vi "0805_Visão_de_máquina_alterado.vi"() -> ()   [LabVIEW 2017]
uses:
  <vilib>/userdefined/High Color/IMAQdx.ctl
  <vilib>/vision/driver/IMAQdx.llb/IMAQdx Acquisition Mode.ctl
  <vilib>/vision/driver/IMAQdx.llb/IMAQdx Buffer Number Mode.ctl
  <vilib>/vision/Classification.llb/IMAQ Classifier Read Options.ctl
  <vilib>/vision/driver/NI_Vision_Acquisition_Software.lvlib
  <vilib>/vision/NI_Vision_Development_Module.lvlib
panel:
  out "String":string="Vermelho"
  in  "largura_y":sgl=30.0
  in  "largura_x":sgl=30.0
  in  "ofset y":sgl
  in  "ofset x":sgl
  out "Local destino":T1(ring)
  in  "Tab Control":T2(tab)
  in  "Cluster A":T3
  in  "Cluster B":T3
  in  "Cluster C":T3
  in  "QRCode":bool
  out "Table":string[][](table)
  in  "Stop 2":bool
  in  "Stop 1":bool
  out "Imagem Original":T4(plugin-control)
  in  "Câmera":T5="cam1"
  out "XY Graph 2":cluster{"X":dbl, "Y":dbl}[](graph)
  # "0"
  # "-250"
  # "400"
  # "80"
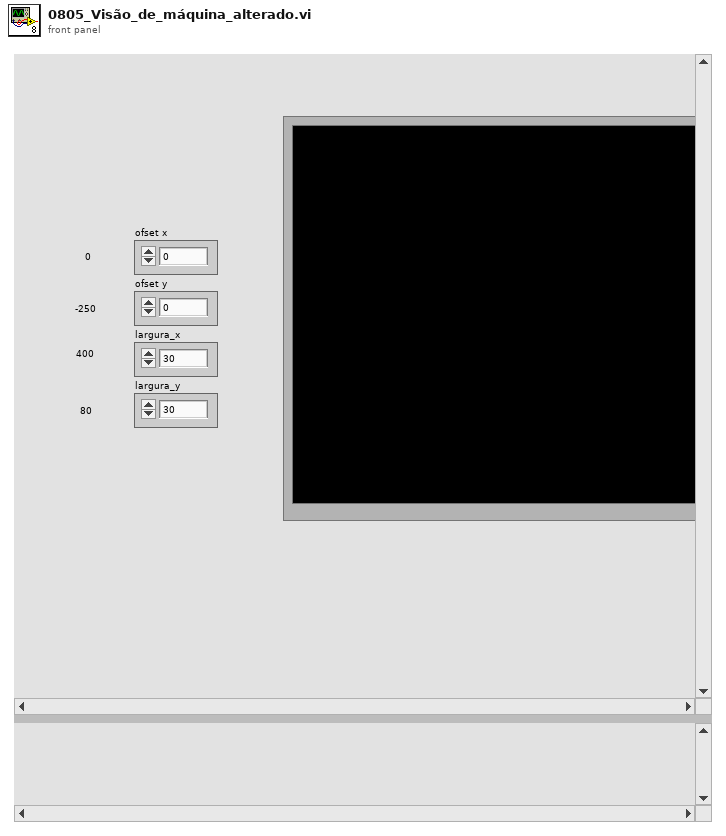
[diagram p1: front panel]
types:
  T1 = enum16{"Local A", "Local B", "Local C", "Discard"}
  T2 = enum32{"Local A", "Local B", "Local C", "QRCode"}
  T3 = cluster{"Azul":bool, "Verde":bool, "Vermelho":bool, "Amarelo":bool, "Quadrado":bool, "Triângulo":bool, "Trapézio":bool}
  T4 = typedef "IMAQ Image.ctl" = refnum<image>
  T5 = typedef "IMAQdx.ctl" = refnum<k21>
  T6 = typedef "NI_Vision_Acquisition_Software.lvlib/IMAQdx Acquisition Mode.ctl" = enum32{"One Shot", "Continuous"}
  T7 = typedef "NI_Vision_Acquisition_Software.lvlib/IMAQdx Buffer Number Mode.ctl" = enum32{"Next", "Last", "Buffer Number", "Every", "Last New"}
  T8 = cluster{"Global Rectangle":i32[], "Contours":cluster{"Contour Type":u32, "ROI Type":u32, "Points":i32[]}[]}
  T9 = typedef "ROI Descriptor" = cluster{"Global Rectangle":i32[], "Contours":cluster{"ID":enum32{"External", "Internal"}, "Type":u32, "Coordinates":i32[]}[]}
  T10 = typedef "IMAQ Classifier Read Options.ctl" = i32
  T11 = typedef "IMAQ Classifier Session.ctl" = refnum<k1>
  T12 = cluster{"Contour Type":u32, "ROI Type":u32, "Points":i32[]}[]
  T13 = cluster{"Contour Type":u32, "ROI Type":u32, "Points":i32[]}
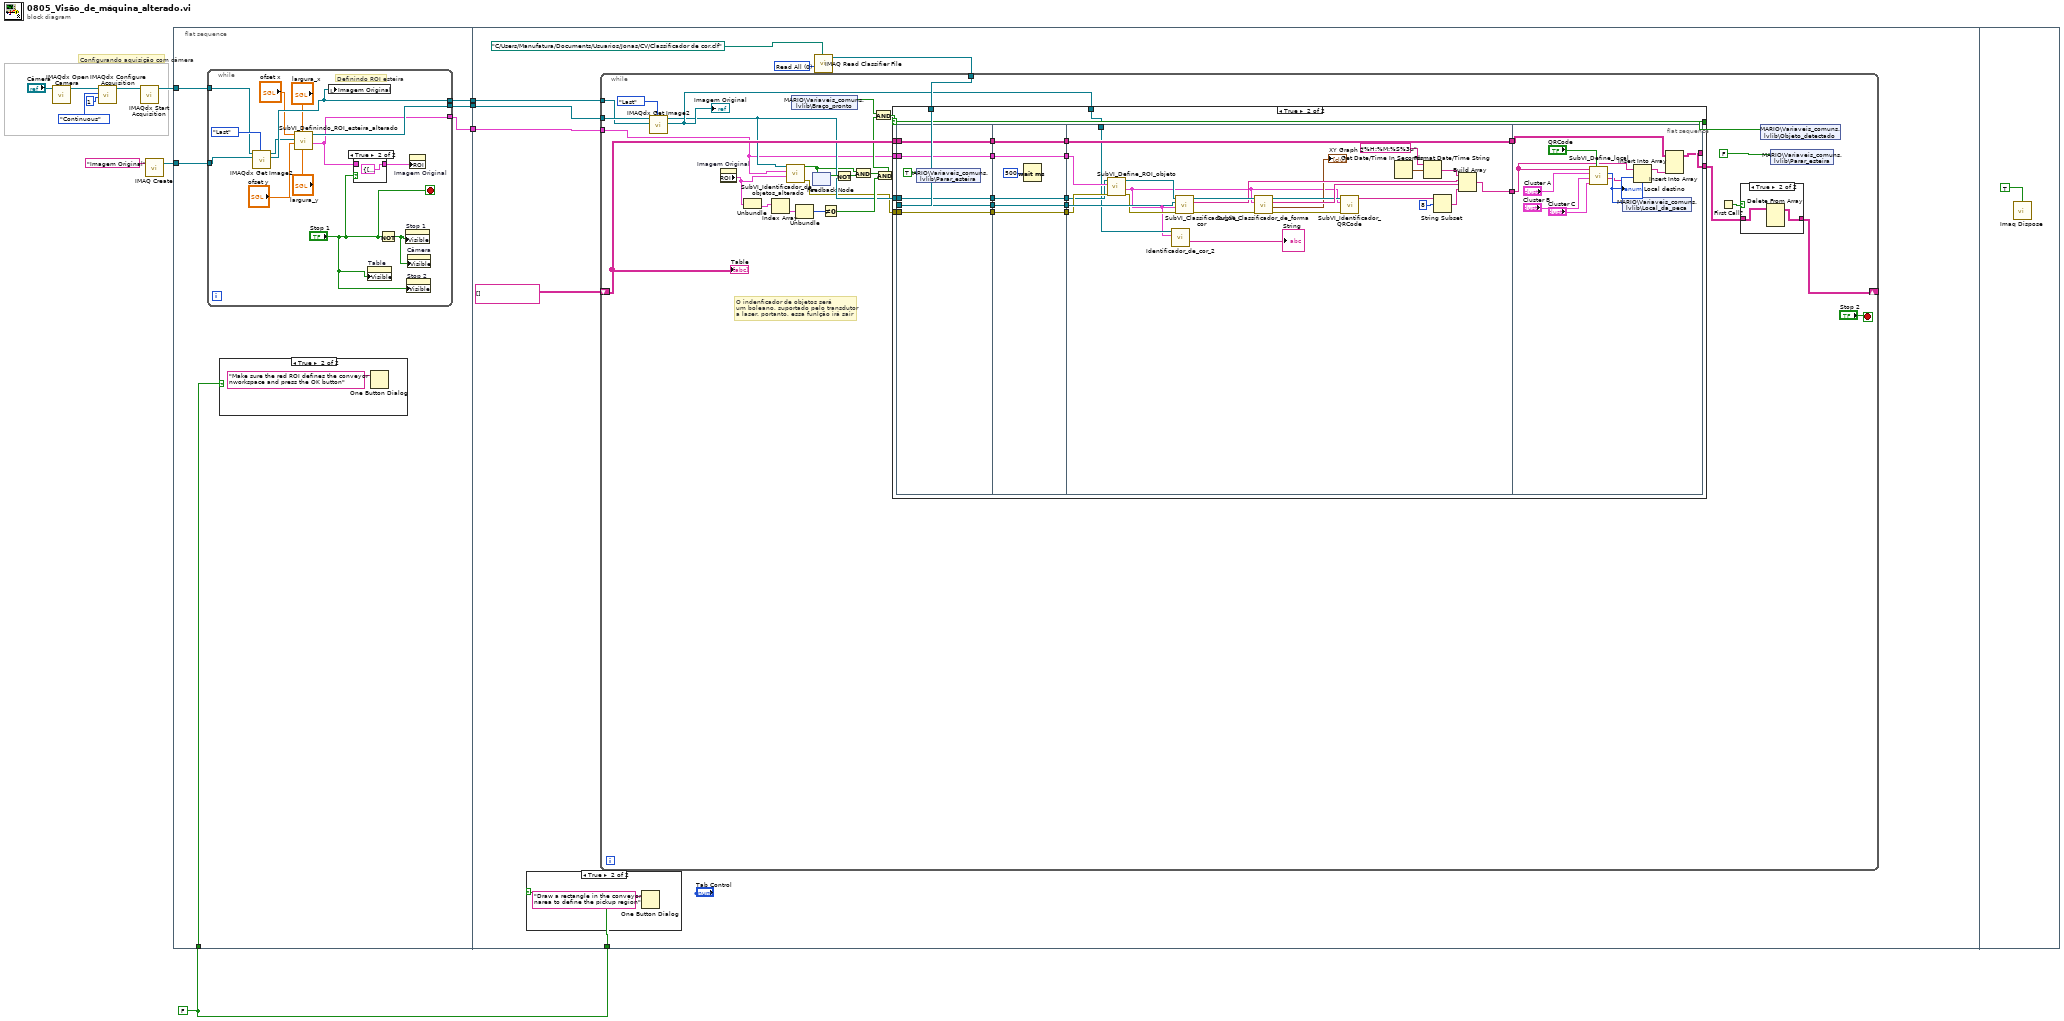
[diagram p0: block diagram]
diagram:
  w1 = FALSE
  # "Configurando aquisição com câmera"
  n1 = call <vilib>:"IMAQdx Open Camera.vi"("Session In"="Câmera") -> ("Session Out"=w12:T5)  [unwired: 9 in, 1 out]
  n2 = call <vilib>:"IMAQdx Configure Acquisition.vi"("Number of Buffers"=u32 1, "Continuous?"=IMAQdx_Acquisition_Mode."Continuous", "Session In"=w12) -> ("Session Out"=w11:T5)  [unwired: 7 in, 1 out]
  n3 = call <vilib>:"IMAQdx Start Acquisition.vi"("Session In"=w11) -> ("Session Out"=w7:T5)  [unwired: 9 in, 1 out]
  n4 = call "IMAQ Create"("Image Name"="Imagem Original") -> ("New Image"=w5:T4)  [unwired: 4 in, 1 out]
  n5 = flat-sequence {
    tunnel: w7 -> [w18]
    tunnel: w5 -> [w17]
    tunnel: [w16] -> w4
    tunnel: [w15] -> w3
    tunnel: [w14] -> w2
    tunnel: w1 -> [w13]
    tunnel: w4 -> [w43]
    tunnel: w3 -> [w42]
    tunnel: w2 -> [w41]
    tunnel: w1 -> [w40]
    frame #0 {
      n6 = while {
        tunnel: w18 -> [w32]
        tunnel: w17 -> [w31]
        tunnel: [w25] -> w16
        tunnel: [w24] -> w15
        tunnel: [w29] -> w14
        stop <- "Stop 1" stop-if-true
        # "Definindo ROI esteira"
        n7 = call <vilib>:"IMAQdx Get Image2.vi"("Buffer Number Mode (Next)"=IMAQdx_Buffer_Number_Mode."Last", "Image In"=w31, "Session In"=w32) -> ("Image Out"=w29:T4, "Session Out"=w26:T5)  [unwired: 5 in, 2 out]
        n8 = call "SubVI_Definindo_ROI_esteira_alterado.vi"("largura_y"="largura_y", "largura_x"="largura_x", "ofset y"="ofset y", "Session in"=w26, "ofset x"="ofset x") -> ("ROI Descriptor"=w24:T9, "Session Out"=w25:T5)  [unwired: 4 in, 1 out]
        n9 = local write "Imagem Original"(w29) -> ()
        n10 = case shown="True" "Stop 1" {
          tunnel: w24 -> [w34 _]
          tunnel: [w34 T8 {"Global Rectangle"=[0, 0, 1, 1], "Contours"=[{"Contour Type"=0, "ROI Type"=1, "Points"=[0, 0]}]} ("ROI")] -> w30
          frame False {
          }
          frame True {
          }
        }
        n11 = property on="Table" class="Tbl (strict)"("Visible"="Stop 1") -> ()  [unwired: 2 in, 2 out]
        n12 = Not(x="Stop 1") -> (.not. x?=w28:bool)
        n13 = property on="Stop 1" class="Bool"("Visible"=w28) -> ()  [unwired: 2 in, 2 out]
        n14 = property on="Stop 2" class="Bool"("Visible"="Stop 1") -> ()  [unwired: 2 in, 2 out]
        n15 = property on="Câmera" class="IMAQdx (strict)"("Visible"=w28) -> ()  [unwired: 2 in, 2 out]
        n16 = property on="Imagem Original" class="ImageControl"("ROI"=w30) -> ()  [unwired: 2 in, 2 out]
      }
      n17 = case shown="True" w13 {
        frame False {
        }
        frame True {
          n18 = One Button Dialog(message="Make sure the red ROI defines the conveyor \nworkspace and press the OK button") -> ()  [unwired: 1 in, 1 out]
        }
      }
    }
    frame #1 {
      w39 = T10 0 items=["Read All", "Add Samples, Do Not Change Options", "Read Options, Do Not Add Samples"] ("Read Options")
      n19 = case shown="True" w40 {
        frame False {
        }
        frame True {
          n20 = One Button Dialog(message="Draw a rectangle in the conveyor\narea to define the pickup region") -> ()  [unwired: 1 in, 1 out]
        }
      }
      n21 = call "IMAQ Read Classifier File"("File Path"=path "C:/Users/Manufatura/Documents/Usuarios/Jonas/CV/Classificador de cor.clf", "Read Options"=w39) -> ("Classifier Session"=w38:T11)  [unwired: 2 in, 7 out]
      n22 = while {
        tunnel: w43 -> [w69]
        tunnel: w42 -> [w47]
        tunnel: w41 -> [w67]
        tunnel: w38 -> [w62]
        shift-right: [w55] -> _
        shift-left: string[][] [] ("Table") -> [w58]
        stop <- "Stop 2" stop-if-true
        # "O indenficador de objetos será\num boleano, suportado pelo transdutor\na laser. portanto, essa funlção irá sair"
        n23 = call <vilib>:"IMAQdx Get Image2.vi"("Buffer Number Mode (Next)"=IMAQdx_Buffer_Number_Mode."Last", "Image In"=w67, "Session In"=w69) -> ("Image Out"=w49:T4, "Session Out"=w48:T5)  [unwired: 5 in, 2 out]
        "Imagem Original" <- w49
        n24 = property on="Imagem Original" class="ImageControl"() -> ("ROI"=w46:T8)  [unwired: 2 in, 2 out]
        n25 = Unbundle(w46) -> ("Contours"=w66:T12)  [unwired: 1 out]
        n26 = Index Array(array=w66) -> (element=w65:T13)  [unwired: 1 in]
        n27 = call "SubVI_Identificador_de_objetos_alterado.vi"("ROI Detecção"=w46, "ROI Esteira"=w47, "Session In"=w48) -> ("error out"=w44:errorcluster, "Objeto Identificado"=w45:bool)  [unwired: 7 in]
        n28 = shared-variable "MARIO\\Variaveis_comuns.lvlib\\Braço_pronto"() -> (w52:bool)  [unwired: 1 in, 1 out]
        n29 = Unbundle(w65) -> ("ROI Type"=w64:u32)  [unwired: 2 out]
        n30 = feedback-in #1(w45) -> ()
        n31 = feedback #1() -> (w60:bool)  [unwired: 1 in]
        n32 = Not Equal To 0?(x=w64) -> (x != 0?=w63:bool)
        n33 = Not(x=w60) -> (.not. x?=w59:bool)
        n34 = And(x=w45, y=w59) -> (x .and. y?=w61:bool)
        n35 = And(x=w61, y=w63) -> (x .and. y?=w51:bool)
        n36 = And(x=w52, y=w51) -> (x .and. y?=w50:bool)
        n37 = case shown="True" w50 {
          selector: w50 -> [w74 w89]
          tunnel: w48 -> [_ w93]
          tunnel: w62 -> [_ w95]
          tunnel: w44 -> [_ w94]
          tunnel: [w75 w92] -> w56
          tunnel: w58 -> [w75 w91]
          tunnel: [w74 w89] -> w54
          tunnel: w47 -> [_ w88]
          tunnel: w49 -> [_ w76]
          frame False {
          }
          frame True {
            n38 = flat-sequence {
              tunnel: w91 -> [w98]
              tunnel: w93 -> [w99]
              tunnel: w94 -> [w100]
              tunnel: w95 -> [w101]
              tunnel: [w101] -> w87
              tunnel: [w100] -> w85
              tunnel: [w99] -> w83
              tunnel: [w98] -> w81
              tunnel: w88 -> [w96]
              tunnel: [w96] -> w79
              tunnel: w87 -> [w107]
              tunnel: [w107] -> w86
              tunnel: w85 -> [w106]
              tunnel: [w106] -> w84
              tunnel: w83 -> [w105]
              tunnel: [w105] -> w82
              tunnel: w81 -> [w104]
              tunnel: [w104] -> w80
              tunnel: w79 -> [w103]
              tunnel: [w103] -> w78
              tunnel: [w119] -> w90
              tunnel: w86 -> [w131]
              tunnel: w84 -> [w116]
              tunnel: w82 -> [w114]
              tunnel: w80 -> [w113]
              tunnel: w78 -> [w117]
              tunnel: [w113] -> w77
              tunnel: w76 -> [w109]
              tunnel: [w135] -> w92
              tunnel: w90 -> [w134]
              tunnel: w77 -> [w136]
              frame #0 {
                n39 = shared-variable "MARIO\\Variaveis_comuns.lvlib\\Parar_esteira"(TRUE ("Parar_esteira")) -> ()  [unwired: 1 in, 1 out]
              }
              frame #1 {
                n40 = Wait (ms)(milliseconds to wait=u32 500) -> ()  [unwired: 1 out]
              }
              frame #2 {
                n41 = call "SubVI_Define_ROI_objeto.vi"("error in (no error)"=w116, "ROI Esteira"=w117, "Session In"=w114) -> ("error out"=w115:errorcluster, "ROI Objeto"=w108:T9, "Session Out"=w110:T5)  [unwired: 5 in, 1 out]
                n42 = call "Identificador_de_cor_2.vi"("ROI Objeto"=w108, "Refnum in"=w109) -> ("String"=→"String":string)  [unwired: 6 in, 3 out]
                n43 = call "SubVI_Classificador_de_cor.vi"("error in"=w115, "ROI Objeto"=w108, "Classifier Session"=w131, "Session In"=w110) -> ("error out"=w130:errorcluster, "Class"=w118:string, "Session Out"=w125:T5)  [unwired: 5 in]
                n44 = call "SubVI_Classificador_de_forma.vi"("error in"=w130, "ROI Objeto"=w108, "Session In"=w125) -> ("error out"=w126:errorcluster, "Points"=→"XY Graph 2":cluster{"X":dbl, "Y":dbl}[], "Forma"=w124:string, "Session Out"=w123:T5)  [unwired: 5 in]
                n45 = call "SubVI_Identificador_QRCode.vi"("error in"=w126, "ROI Objeto"=w108, "Session In"=w123) -> ("Data"=w122:string)  [unwired: 7 in, 1 out]
                n46 = Get Date/Time In Seconds() -> (seconds since 1Jan1904=w128:timestamp)
                n47 = Format Date/Time String(time format string (%c)="%H:%M:%S%3u", seconds (now)=w128) -> (date/time string=w127:string)  [unwired: 1 in]
                n48 = String Subset(string=w122, offset (0)=8) -> (substring=w121:string)  [unwired: 1 in]
                n49 = Build Array(w127, w118, w124, w121) -> (w119:string[])
              }
              frame #3 {
                n50 = call "SubVI_Define_local.vi"("QRCode"="QRCode", "Cluster C"="Cluster C", "Cluster B"="Cluster B", "Cluster A"="Cluster A", "Linha da tabela"=w134) -> ("Destino"=w132:string, "Local destino"=w138:T1)  [unwired: 5 in]
                "Local destino" <- w138
                n51 = shared-variable "MARIO\\Variaveis_comuns.lvlib\\Local_da_peca"(w138) -> ()  [unwired: 1 in, 1 out]
                n52 = Insert Into Array(array=w134, new element=w132) -> (w133:string[])  [unwired: 1 in]
                n53 = Insert Into Array(array=w136, new element=w133) -> (w135:string[][])  [unwired: 2 in]
              }
            }
          }
        }
        n54 = First Call?() -> (First Call?: T/F=w57:bool)
        n55 = case shown="True" w57 {
          tunnel: w56 -> [w71 w73]
          tunnel: [w71 w72] -> w55
          frame False {
          }
          frame True {
            n56 = Delete From Array(array=w73) -> (array with subset deleted=w72:string[][])  [unwired: 3 in, 1 out]
          }
        }
        n57 = shared-variable "MARIO\\Variaveis_comuns.lvlib\\Objeto_detectado"(w54) -> ()  [unwired: 1 in, 1 out]
        n58 = shared-variable "MARIO\\Variaveis_comuns.lvlib\\Parar_esteira"(FALSE ("Parar_esteira")) -> ()  [unwired: 1 in, 1 out]
        "Table" <- w58
      }
    }
    frame #2 {
      n59 = call "Imaq Dispose"("All Images? (No)"=TRUE) -> ()  [unwired: 5 in, 1 out]
    }
  }
